vi "Add Reporter.vi"(8 "error in (no error)":errorcluster, 10 "Reporter to Add":refnum<class "Reporter.lvclass">, 11 "Report With First Working in":refnum<class "Report With First Working.lvclass">) -> (0 "error out":errorcluster, 3 "Report With First Working out":refnum<class "Report With First Working.lvclass">)   [LabVIEW 2020]
uses:
  Report With First Working.lvclass/Report With First Working.ctl
  Report With First Working.lvclass
  Reporter/Reporter.lvclass
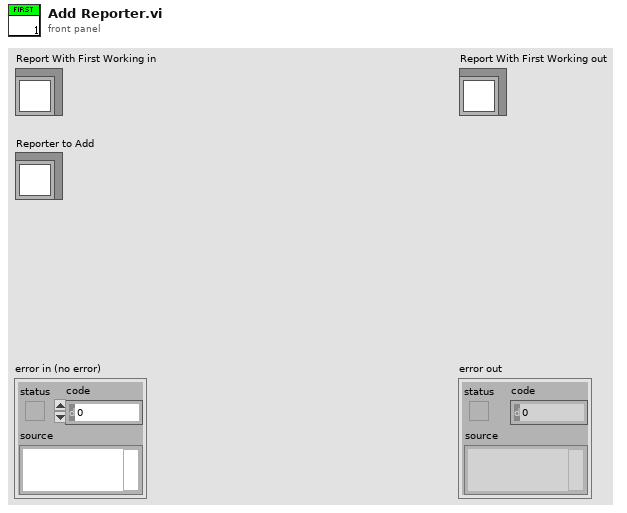
[diagram p1: front panel]
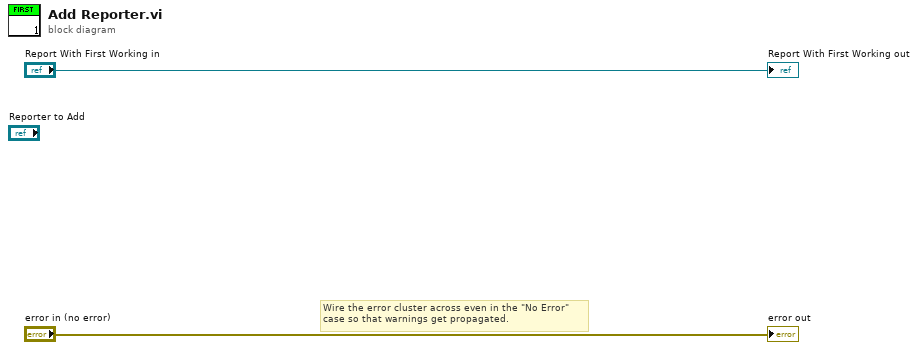
[diagram p0: block diagram]
diagram:
  # "Wire the error cluster across even in the \"No Error\"\ncase so that warnings get propagated."
  "error out" <- "error in (no error)"
  "Report With First Working out" <- "Report With First Working in"
